vi "Log in.vi"(8 "error in":errorcluster, 10 "String in":string, 11 "Refnum in":T1) -> (0 "error out":errorcluster, 1 "String out":string, 2 "Enum":T2=enum."Initial", 3 "Refnum out":T1, 4 "T/F":bool)   [LabVIEW 2017]
uses:
  Control/State machine.ctl
  <vilib>/addons/database/Connection.llb/Conn ObjectReference.ctl
  <vilib>/addons/database/_DB Variant To Data/Database Variant To Data.xnode
  <vilib>/addons/database/NI_Database_API.lvlib
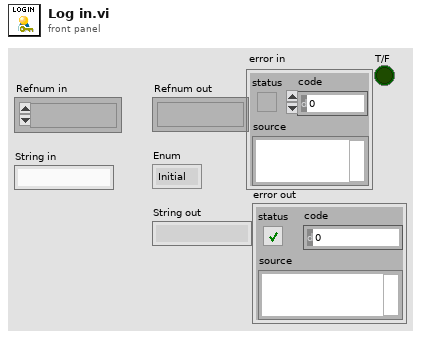
[diagram p1: front panel]
types:
  T1 = typedef "NI_Database_API.lvlib/Conn ObjectReference.ctl" = refnum<k1>
  T2 = typedef "State machine.ctl" = enum16{"Licence check", "Initial", "Log in", "Creat Config file", "Network setting", "Creat database 1", "Creat database 2", "Creat database 3", "Transfer", "Begin", "Exit"}
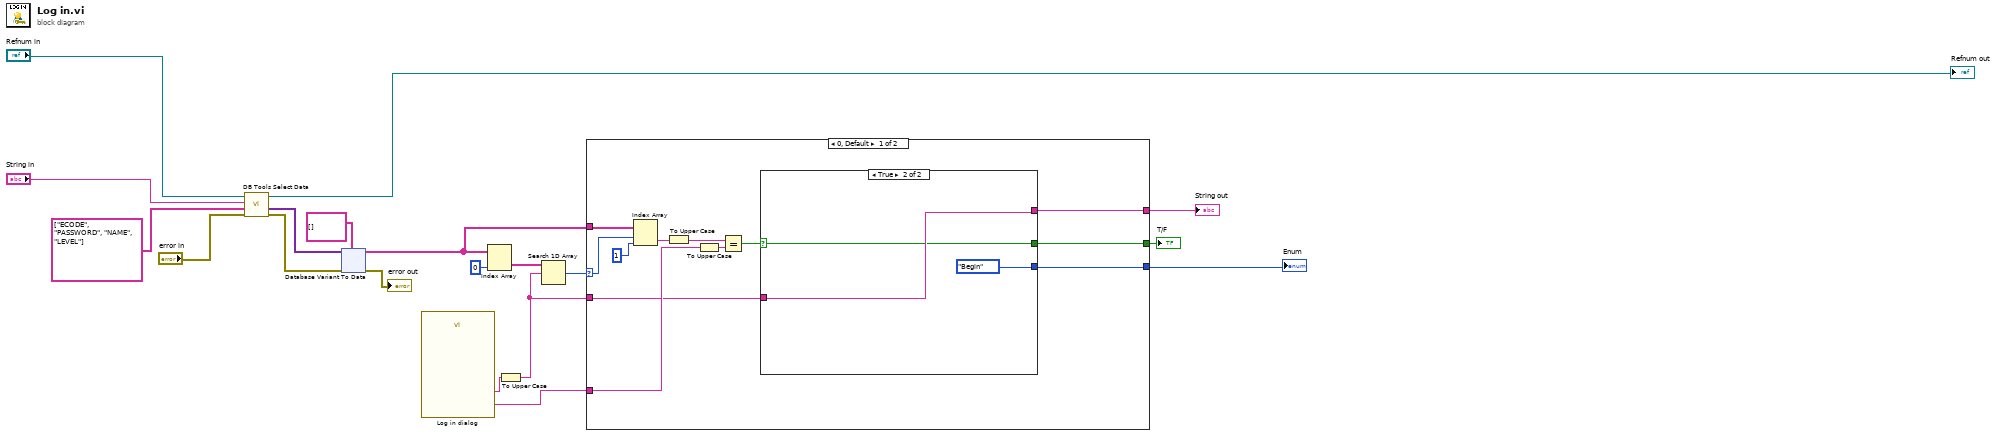
[diagram p0: block diagram]
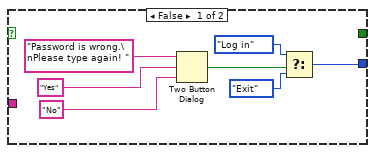
[diagram p2: hidden frame]
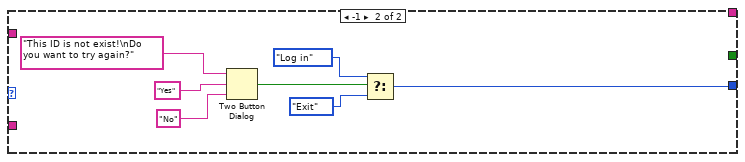
[diagram p3: hidden frame]
diagram:
  n1 = call <vilib>:"DB Tools Select Data.vi"("error in (no error)"="error in", "columns"=string[] ["ECODE", "PASSWORD", "NAME", "LEVEL"], "table"="String in", "connection reference"="Refnum in") -> ("error out"=w4:errorcluster, "data"=w9:variant[][], "connection reference out"=→"Refnum out":T1)  [unwired: 2 in]
  n2 = xnode "Database Variant To Data"("database variant"=w9, "error in (no error)"=w4, "type"=string[][] []) -> ("data"=w15:string[][], "error out"=→"error out":errorcluster)
  n3 = call "Log in dialog.vi"() -> ("Password"=w16:string, "ID"=w13:string)  [unwired: 16 in, 2 out]
  n4 = Index Array(array=w15, index (col)=0 ("disabled index (col)")) -> (element=w12:string[])  [unwired: 1 in]
  n5 = To Upper Case(1:w13) -> (0:w19:string)
  n6 = Search 1D Array(1D array=w12, element=w19) -> (index of element=w14:i32)  [unwired: 1 in]
  n7 = case shown="0, Default" w14 {
    selector: w14 -> [w30 _]
    tunnel: [w25 w42] -> w17
    tunnel: w15 -> [w31 _]
    tunnel: w16 -> [w27 _]
    tunnel: [w22 _] -> w18
    tunnel: w19 -> [w21 _]
    tunnel: [w20 _] -> w1
    frame 0, Default {
      n8 = Index Array(array=w31, index (row)=w30, index (col)=1 ("disabled index (col)")) -> (element=w28:string)
      n9 = To Upper Case(1:w28) -> (0:w23:string)
      n10 = To Upper Case(1:w27) -> (0:w24:string)
      n11 = Equal?(x=w23, y=w24) -> (x = y?=w26:bool)
      n12 = case shown="True" w26 {
        selector: w26 -> [_ w39]
        tunnel: [w32 State_machine."Begin" ("Enum")] -> w25
        tunnel: [_ w40] -> w22
        tunnel: w21 -> [_ w40]
        tunnel: [_ w39] -> w20
        frame False {
          n13 = Two Button Dialog(message="Password is wrong.\nPlease type again! ", 1:"No" ("T button name (\"OK\")"), 2:"Yes" ("T button name (\"OK\")")) -> (T button?=w35:bool)
          n14 = Select(t=State_machine."Log in" ("Enum"), s=w35, f=State_machine."Exit" ("Enum")) -> (s? t:f=w32:T2)
        }
        frame True {
        }
      }
    }
    frame -1 {
      n15 = Two Button Dialog(message="This ID is not exist!\nDo you want to try again?", 1:"No" ("F button name (\"Cancel\")"), 2:"Yes" ("T button name (\"OK\")")) -> (T button?=w45:bool)
      n16 = Select(t=State_machine."Log in" ("Enum"), s=w45, f=State_machine."Exit" ("Enum")) -> (s? t:f=w42:T2)
    }
  }
  "String out" <- w18
  "Enum" <- w17
  "T/F" <- w1
